vi "Tree.Set.Pass.vi"(8 "error in (no error)":errorcluster, 9 "Edit Tree Items:Add Item":string, 10 "Passed":bool, 11 "TreeControl in":refnum<vi>) -> (0 "error out":errorcluster, 3 "TreeControl out":refnum<vi>)   [LabVIEW 2015, in "Analysis.lvlib"]
uses:
  Analysis.lvlib
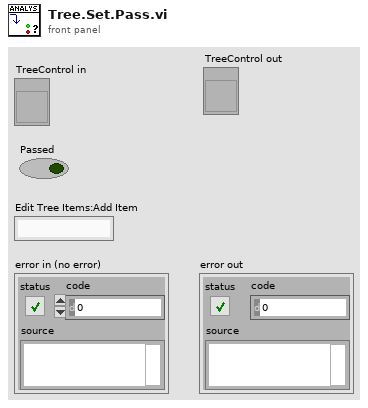
[diagram p1: front panel]
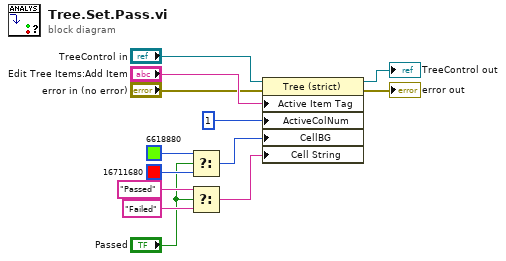
[diagram p0: block diagram]
diagram:
  n1 = Select(t=u32 6618880, s="Passed", f=u32 16711680) -> (s? t:f=w6:u32)
  n2 = Select(t="Passed", s="Passed", f="Failed") -> (s? t:f=w7:string)
  n3 = property class="Tree (strict)"(reference="TreeControl in", error in="error in (no error)", "Active Item Tag"="Edit Tree Items:Add Item", "ActiveColNum"=1 ("Active Cell:Active Column Number"), "CellBG"=w6, "Cell String"=w7) -> (reference out=→"TreeControl out":refnum<vi>, error out=→"error out":errorcluster)
